vi "Close.vi"(8 "error in":errorcluster, 11 "DAQmx BufferLastReadsDBL in":refnum<class "DAQmx BufferLastReadsDBL.lvclass">) -> (0 "error out":errorcluster, 3 "DAQmx BufferLastReadsDBL out":refnum<class "DAQmx BufferLastReadsDBL.lvclass">)   [LabVIEW 2023, in "DAQmx BufferLastReadsDBL.lvclass"]
uses:
  DAQmx BufferLastReadsDBL.lvclass
  DAQmx BufferLastReadsDBL.lvclass/DAQmx BufferLastReadsDBL.ctl
  DAQmx Base CFG/DAQmx Base CFG.lvclass
  BufferLastReadingsDBL/BufferLastReadsDBL.lvclass
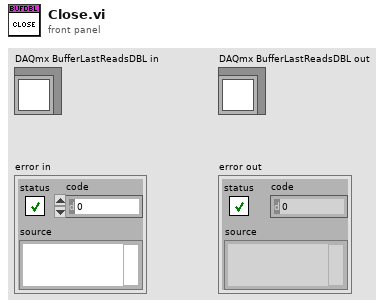
[diagram p1: front panel]
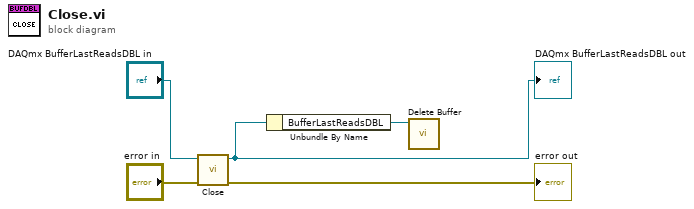
[diagram p0: block diagram]
diagram:
  n1 = call-parent "Close.vi"("error in"="error in", "DAQmx Base CFG in"="DAQmx BufferLastReadsDBL in") -> ("error out"=→"error out":errorcluster, "DAQmx Base CFG out"=w1:refnum<class "DAQmx BufferLastReadsDBL.lvclass">)  [unwired: 8 in]
  "DAQmx BufferLastReadsDBL out" <- w1
  n2 = Unbundle By Name(w1) -> ("BufferLastReadsDBL"=w4:refnum<class "BufferLastReadsDBL.lvclass">)
  n3 = call "Delete Buffer.vi"("BufferLastReadings DBL in"=w4) -> ()  [unwired: 10 in, 1 out]
